vi "Replace Backslash Codes by Special Characters.vi"(2 "String (\\n)":string) -> (7 "String (\\\\n)":string)   [LabVIEW 2021, in "Strings.lvlib"]
uses:
  Strings.lvlib
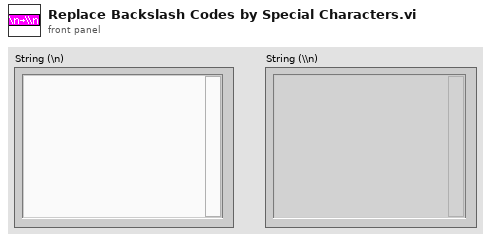
[diagram p1: front panel]
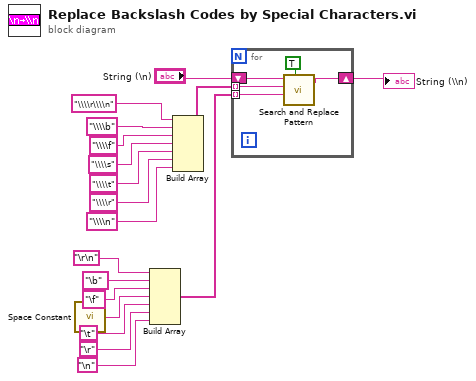
[diagram p0: block diagram]
diagram:
  n1 = call <vilib>:"Space Constant.vi"() -> ("String"=w18:string)
  n2 = Build Array("\r\n", "\b" ("element"), "\f" ("element"), w18, "\t", "\r", "\n") -> (w4:string[])
  n3 = Build Array("\\\\r\\\\n" ("element"), "\\\\b" ("element"), "\\\\f" ("element"), "\\\\s" ("element"), "\\\\t" ("element"), "\\\\r" ("element"), "\\\\n" ("element")) -> (w5:string[])
  n4 = for {
    tunnel: w5 -> [w22] mode=indexing
    tunnel: w4 -> [w21] mode=indexing
    shift-right: [w20] -> w3
    shift-left: "String (\\n)" -> [w23]
    n5 = call <vilib>:"Search and Replace Pattern.vi"("string"=w23, "regular expression (\"\")"=w22, "replace string (\"\")"=w21, "replace all? (F)"=TRUE) -> ("result string"=w20:string)  [unwired: 1 in, 1 out]
  }
  "String (\\\\n)" <- w3
